vi "Read DemodSubCarr.vi"(8 "error in (no error)":errorcluster, 11 "Store in":refnum<class "Store.lvclass">) -> (0 "error out":errorcluster, 2 "DemodSubCarr":waveform(cdb), 3 "Store out":refnum<class "Store.lvclass">)   [LabVIEW 2019, in "Store.lvclass"]
uses:
  Store.lvclass
  Store.lvclass/Store.ctl
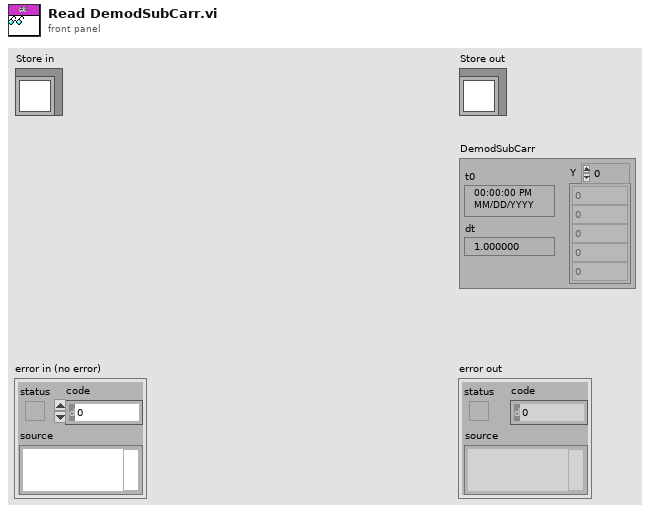
[diagram p1: front panel]
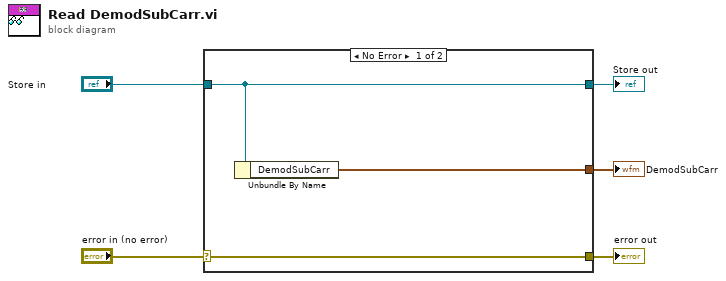
[diagram p0: block diagram]
diagram:
  n1 = case shown="No Error" "error in (no error)" {
    selector: "error in (no error)" -> [w8 w9]
    tunnel: [w8 w9] -> w4
    tunnel: [w7 w10] -> w2
    tunnel: "Store in" -> [w7 w10]
    tunnel: [w6 _] -> w1
    frame No Error {
      n2 = Unbundle By Name(w7) -> ("DemodSubCarr"=w6:waveform(cdb))
    }
    frame Error {
    }
  }
  "error out" <- w4
  "Store out" <- w2
  "DemodSubCarr" <- w1
